vi "resize screen.vi"(0 "This VI":refnum<vi>) -> ()   [LabVIEW 2020, in "Popup Dialog.lvlib"]
uses:
  Popup Dialog.lvlib
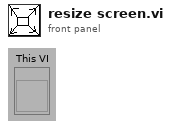
[diagram p1: front panel]
types:
  T1 = cluster{"Left":i16, "Top":i16, "Right":i16, "Bottom":i16}
  T2 = typedef "LVAllMonitorsDisplayTypeDef.ctl" = cluster{"Bounds":cluster{"Left":i16, "Top":i16, "Right":i16, "Bottom":i16}, "Depth":i16}[]
  T3 = cluster{"Bounds":cluster{"Left":i16, "Top":i16, "Right":i16, "Bottom":i16}, "Depth":i16}
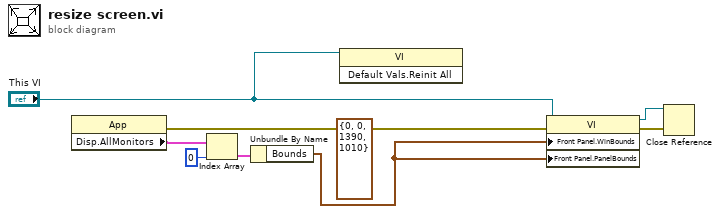
[diagram p0: block diagram]
diagram:
  (unwired) T1 {"Left"=0, "Top"=0, "Right"=1390, "Bottom"=1010} ("Bounds")
  n1 = property class="App"() -> (error out=w5:errorcluster, "Disp.AllMonitors"=w8:T2)  [unwired: 2 in, 1 out]
  n2 = Index Array(array=w8, index=0) -> (element=w7:T3)
  n3 = Unbundle By Name(w7) -> ("Bounds"=w2:T1)
  n4 = invoke class="VI" method="Default Vals.Reinit All"(reference="This VI") -> ()  [unwired: 2 in, 3 out]
  n5 = property class="VI"(reference="This VI", error in=w5, "Front Panel.WinBounds"=w2, "Front Panel.PanelBounds"=w2) -> (reference out=w3:refnum<vi>, error out=w4:errorcluster)
  n6 = Close Reference(reference=w3, error in (no error)=w4) -> ()  [unwired: 1 out]
